vi "readneval_LockIn.vi"(6 "error in":errorcluster, 8 "Handle In":T1 {"Conn" format="0x%08x"}) -> (0 "Theta reference":dbl, 1 "Error Out":errorcluster, 2 "R reference":dbl, 3 "R signal":dbl, 4 "Handle Out":T1 {"Conn" format="0x%08x"}, 5 "Theta signal":dbl, 7 "Freq (Hz)":dbl)   [LabVIEW 2014]
uses:
  <instrlib>/Zurich Instruments LabOne/Public/ziTypeHandle.ctl
  <instrlib>/Zurich Instruments LabOne/Zurich Instruments LabOne.lvlib
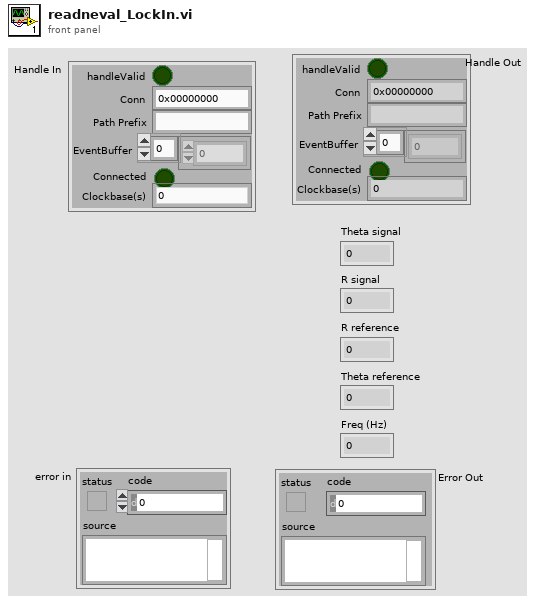
[diagram p1: front panel]
types:
  T1 = typedef "Zurich Instruments LabOne.lvlib/ziTypeHandle.ctl" = cluster{"handleValid":bool, "Conn":u64, "Path Prefix":string, "EventBuffer":u8[], "Connected":bool, "Clockbase(s)":dbl}
  T2 = cluster{"Timestamps (ticks)":u64, "X (Vrms)":dbl, "Y (Vrms)":dbl, "Osc Phase (deg)":dbl, "Freq (Hz)":dbl, "DIO":u32, "AuxIn0 (V)":dbl, "AuxIn1 (V)":dbl}
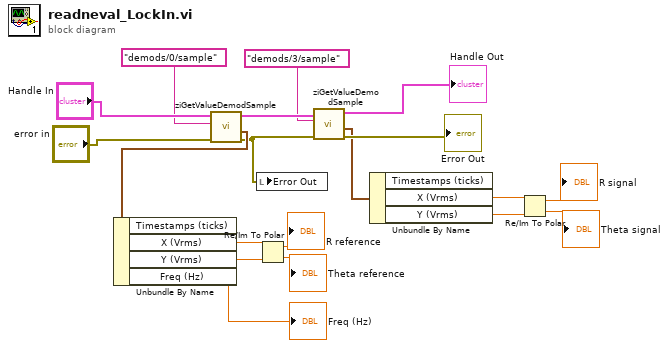
[diagram p0: block diagram]
diagram:
  n1 = call <instrlib>:"ziGetValueDemodSample.vi"("error in"="error in", "Path"="demods/0/sample", "Handle In"="Handle In") -> ("error out"=w6:errorcluster, "Demod Sample Out"=w13:T2, "Handle Out"=w17:T1)  [unwired: 2 in]
  n2 = Unbundle By Name(w13) -> ("X (Vrms)"=w11:dbl, "Y (Vrms)"=w10:dbl, "Freq (Hz)"=→"Freq (Hz)":dbl)  [unwired: 1 out]
  n3 = local write "Error Out"(w6) -> ()
  n4 = Re/Im To Polar(2:w10, 3:w11) -> (0:→"Theta reference":dbl, 1:→"R reference":dbl)
  n5 = call <instrlib>:"ziGetValueDemodSample.vi"("error in"=w6, "Path"="demods/3/sample", "Handle In"=w17) -> ("error out"=→"Error Out":errorcluster, "Demod Sample Out"=w12:T2, "Handle Out"=→"Handle Out":T1)  [unwired: 2 in]
  n6 = Unbundle By Name(w12) -> ("X (Vrms)"=w9:dbl, "Y (Vrms)"=w8:dbl)  [unwired: 1 out]
  n7 = Re/Im To Polar(2:w8, 3:w9) -> (0:→"Theta signal":dbl, 1:→"R signal":dbl)
